vi "Services.Compile.vi"(8 "error in (no error)":errorcluster, 11 "Section Ref in":T4 format="%.0x") -> (0 "error out":errorcluster, 2 "Settings":T1[](array[typedef]) {"Signal.Cmd.Refs"."Signal Refs" format="%.0x"; "Signal.Cmd.Info"."Signals"."Byte Order" items=["Little Endian", "Big Endian"]; "Signal.Cmd.Info"."Signals"."Data Type" items=["Signed", "Unsigned", "IEEE Float"]; "Settings.Refs"."Signal Refs" format="%.0x"; "Signal.Resp.Refs"."Signal Refs" format="%.0x"; "Signal.Resp.Info"."Signals"."Byte Order" items=["Little Endian", "Big Endian"]; "Signal.Resp.Info"."Signals"."Data Type" items=["Signed", "Unsigned", "IEEE Float"]; "Trigger.Refs"."Signal Refs" format="%.0x"; "Status.Refs"."Signal Refs" format="%.0x"}, 3 "Section Ref out":T4 format="%.0x")   [LabVIEW 2019, in "Diagnostics Addon System Explorer.lvlib"]
uses:
  Diagnostics Addon System Explorer.lvlib
  <vilib>/NI VeriStand/Custom Device Tools/Custom Device Utility Library/Custom Device Utility Library.lvlib
  Types/Frame.Ref.ctl
  Types/FG.Action.ctl
  <vilib>/NI VeriStand/Custom Device API/Custom Device Item Ref.ctl
  <vilib>/NI VeriStand/Custom Device API/Custom Device API.lvlib
  Shared/Types/Signal.ctl
  Shared/Diagnostics Addon Shared.lvlib
  Shared/Types/Frame.Compile.ctl
  Shared/Types/Type.ctl
  Types/Service.Export.ctl
  <vilib>/NI VeriStand/Custom Device Tools/Custom Device Utility Library/NI VeriStand - Search for Item by GUID.vi
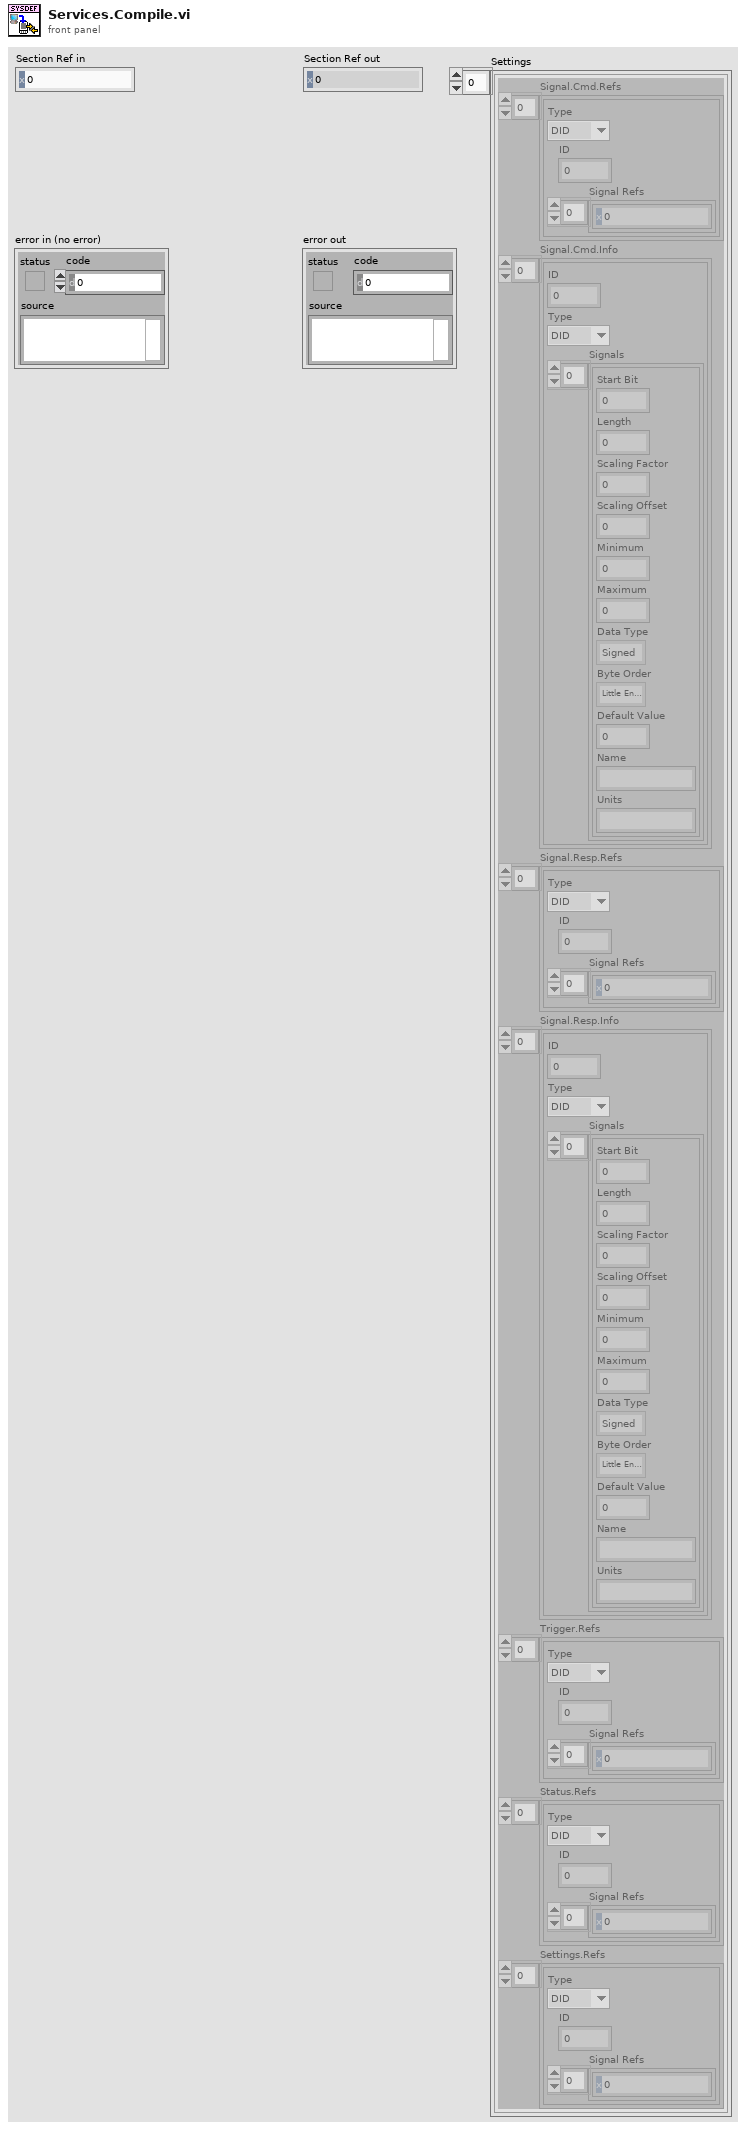
[diagram p1: front panel]
types:
  T1 = typedef "Diagnostics Addon System Explorer.lvlib/Service.Export.ctl" = cluster{"Signal.Cmd.Refs":T2[], "Signal.Cmd.Info":T5[], "Signal.Resp.Refs":T2[], "Signal.Resp.Info":T5[], "Trigger.Refs":T2[], "Status.Refs":T2[], "Settings.Refs":T2[]}
  T2 = typedef "Diagnostics Addon System Explorer.lvlib/Frame.Ref.ctl" = cluster{"Type":T3, "ID":u32, "Signal Refs":T4[]}
  T3 = typedef "Diagnostics Addon Shared.lvlib/Type.ctl" = enum16{"DID", "CDID", "PID", "CPID", "Read Memory", "Write Memory", "IO Control", "Routine Start", "Routine Request", "Routine Stop", "User Defined", "DTC Control", "Clear DTCs", "Read DTCs", "Start DTCs", "DTC Change Count", "Tester Present", "Unlock ECU", "Reset ECU", "Diag Session Control", "Communication Control", "DPID Control", "Poll Control", "Diag CAN Control"}
  T4 = typedef "Custom Device API.lvlib/Custom Device Item Ref.ctl" = u64
  T5 = typedef "Diagnostics Addon Shared.lvlib/Frame.Compile.ctl" = cluster{"ID":u32, "Type":T3, "Signals":T6[]}
  T6 = typedef "Diagnostics Addon Shared.lvlib/Signal.ctl" = cluster{"Start Bit":u32, "Length":u32, "Scaling Factor":dbl, "Scaling Offset":dbl, "Minimum":dbl, "Maximum":dbl, "Data Type":u32, "Byte Order":u32, "Default Value":dbl, "Name":string, "Units":string}
  T7 = typedef "Diagnostics Addon System Explorer.lvlib/FG.Action.ctl" = enum16{"Get", "Set"}
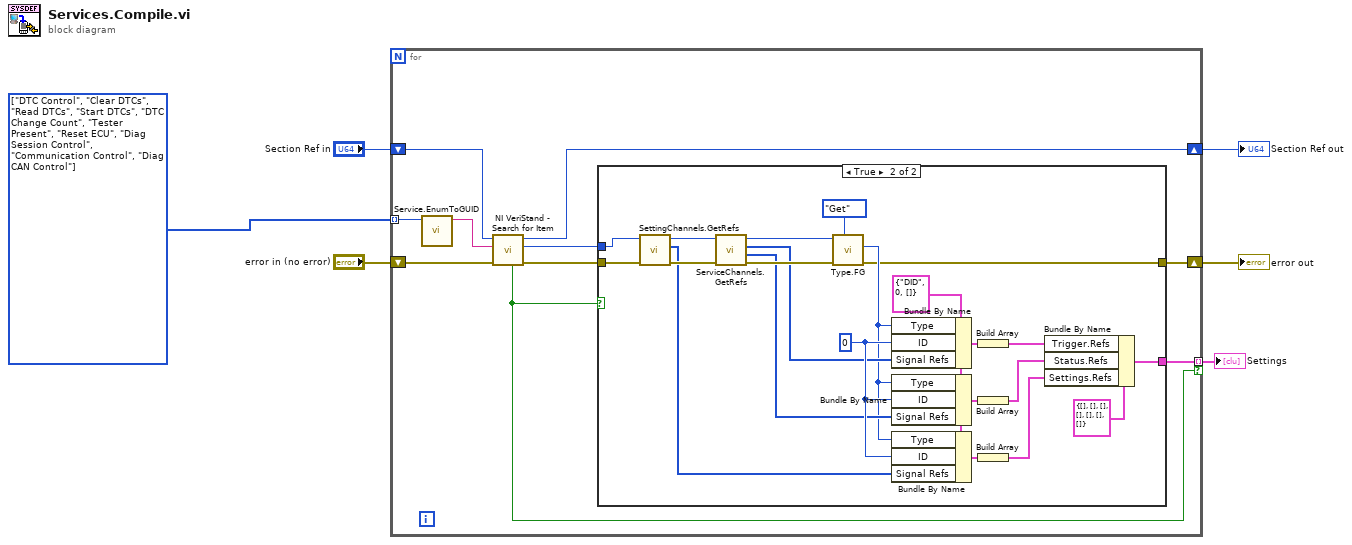
[diagram p0: block diagram]
diagram:
  w1 = T3[] [enum."DTC Control", enum."Clear DTCs", enum."Read DTCs", enum."Start DTCs", enum."DTC Change Count", enum."Tester Present", enum."Reset ECU", enum."Diag Session Control", enum."Communication Control", enum."Diag CAN Control"] items=["DID", "CDID", "PID", "CPID", "Read Memory", "Write Memory", "IO Control", "Routine Start", "Routine Request", "Routine Stop", "User Defined", "DTC Control", "Clear DTCs", "Read DTCs", "Start DTCs", "DTC Change Count", "Tester Present", "Unlock ECU", "Reset ECU", "Diag Session Control", "Communication Control", "DPID Control", "Poll Control", "Diag CAN Control"]
  n1 = for {
    tunnel: [w10] -> w2 mode=indexing if=w9
    shift-right: [w12] -> w4
    shift-left: "Section Ref in" -> [w14]
    shift-right: [w11] -> w3
    shift-left: "error in (no error)" -> [w13]
    tunnel: w1 -> [w7] mode=indexing
    n2 = call "Service.EnumToGUID.vi"("Type"=w7) -> ("GUID"=w8:string)  [unwired: 10 in]
    n3 = call-poly <vilib>:"NI VeriStand - Search for Item.vi"("error in"=w13, "Item GUID"=w8, "Section Ref in"=w14) -> ("error out"=w15:errorcluster, "Item Ref"=w16:T4, "Section Ref out"=w12:T4, "Found"=w9:bool)  [unwired: 5 in]
    n4 = case shown="True" w9 {
      tunnel: [w17 w18] -> w11
      tunnel: w16 -> [_ w31]
      tunnel: w15 -> [w17 w33]
      tunnel: [_ w37] -> w10
      frame False {
      }
      frame True {
        w27 = 0
        w26 = T2 {"Type"=enum."DID", "ID"=0, "Signal Refs"=[]} ("cluster")
        n5 = call "SettingChannels.GetRefs.vi"("error in (no error)"=w33, "Item Ref in"=w31) -> ("error out"=w36:errorcluster, "Settings"=w23:T4[], "Section Ref out"=w35:T4)  [unwired: 7 in]
        n6 = call "ServiceChannels.GetRefs.vi"("error in (no error)"=w36, "Item Ref in"=w35) -> ("error out"=w34:errorcluster, "Status"=w24:T4[], "Trigger"=w25:T4[], "Section Ref out"=w32:T4)  [unwired: 6 in]
        n7 = call "Type.FG.vi"("Action"=FG.Action."Get", "error in (no error)"=w34, "Device Item Ref in"=w32) -> ("error out"=w18:errorcluster, "Type"=w19:T3)  [unwired: 6 in, 1 out]
        n8 = Bundle By Name(cluster=w26, "Type"=w19, "ID"=w27, "Signal Refs"=w25) -> (w30:T2)
        n9 = Bundle By Name(cluster=w26, "Type"=w19, "ID"=w27, "Signal Refs"=w24) -> (w29:T2)
        n10 = Bundle By Name(cluster=w26, "Type"=w19, "ID"=w27, "Signal Refs"=w23) -> (w28:T2)
        n11 = Build Array(w30) -> (w22:T2[])
        n12 = Build Array(w29) -> (w21:T2[])
        n13 = Build Array(w28) -> (w20:T2[])
        n14 = Bundle By Name(cluster=T1 {"Signal.Cmd.Refs"=[], "Signal.Cmd.Info"=[], "Signal.Resp.Refs"=[], "Signal.Resp.Info"=[], "Trigger.Refs"=[], "Status.Refs"=[], "Settings.Refs"=[]}, "Trigger.Refs"=w22, "Status.Refs"=w21, "Settings.Refs"=w20) -> (w37:T1)
      }
    }
  }
  "Section Ref out" <- w4
  "error out" <- w3
  "Settings" <- w2
